vi "Memory.Pointer.Read Bytes.Subset.In Place.Unsafe.vi"(7 "length":u64=18446744073709551615 format="%d bytes", 8 "error in (no error)":errorcluster, 9 "offset (0)":u64 format="%d bytes", 10 "buffer in":u8[](array[numeric]) format="%02x", 11 "Pointer in":refnum<class "Memory.Pointer.lvclass">) -> (0 "error out":errorcluster, 1 "offset dup":u64 format="%d bytes", 2 "buffer out":u8[](array[numeric]) format="%02x", 3 "Pointer out":refnum<class "Memory.Pointer.lvclass">)   [LabVIEW 2016, in "LabVIEW Memory Manager.lvlib" / "Memory.Pointer.lvclass"]
uses:
  Memory.Pointer.lvclass
  Memory.Pointer.lvclass/Memory.Pointer.ctl
  Memory.Pointer.Offset to Address.Unsafe.vi
  Memory.Pointer.Get Address.vi
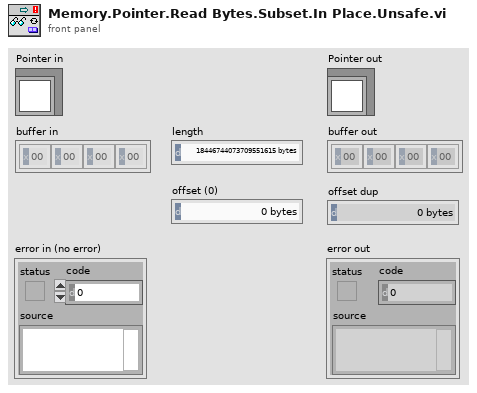
[diagram p1: front panel]
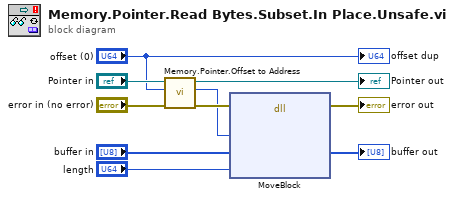
[diagram p0: block diagram]
diagram:
  n1 = call-poly "Memory.Pointer.Offset to Address.vi"("error in (no error)"="error in (no error)", "offset"="offset (0)", "Pointer in"="Pointer in") -> ("error out"=w6:errorcluster, "address"=w5:u64, "Pointer out"=→"Pointer out":refnum<class "Memory.Pointer.lvclass">)  [unwired: 6 in]
  n2 = dll-call lib="LabVIEW" fn="MoveBlock"(error in=w6, "src pointer"=w5, "dst pointer"="buffer in", "size"="length") -> (error out=→"error out":errorcluster, "dst pointer"=→"buffer out":u8[])  [unwired: 5 in, 1 out]
  "offset dup" <- "offset (0)"
